vi "Exemple_Metrics_Label_Ranking_Average_Precision_Score.vi"() -> ()   [LabVIEW 2020]
uses:
  Objet/3 - Model selection and evaluation/3.3 - Metrics and scoring/label_ranking_average_ps/Label_Ranking_Average_PS.vi
panel:
  out "Score":string
  out "error out":errorcluster caption="sortie d'erreur"
  in  "error in (no error)":errorcluster caption="entrée d'erreur (pas d'erreur)"
  in  "label_ranking_average_precision_score":cluster{"sample_weight":dbl[]}
  in  "y_score":string[][](array[string])=[["0,75", "0,5", "1"], ["1", "0,2", "0,1"]]
  in  "y_true":string[][](array[string])=[["1", "0", "0"], ["0", "0", "1"]]
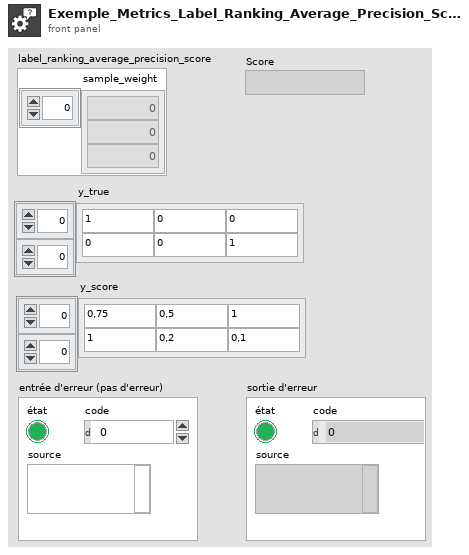
[diagram p1: front panel]
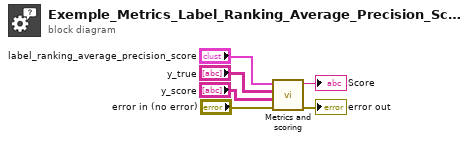
[diagram p0: block diagram]
diagram:
  n1 = call-poly "Metrics and scoring.vi"("error in (no error)"="error in (no error)", "y_score"="y_score", "y_true"="y_true", "label_ranking_average_precision_score"="label_ranking_average_precision_score") -> ("error out"=→"error out":errorcluster, "Score"=→"Score":string)  [unwired: 6 in]
